vi "Uncert Table Layout.vi"(11 "Uncert In":dbl[][](array[numeric])) -> (3 "Uncert Table":string[][](array[string]))   [LabVIEW 2014]
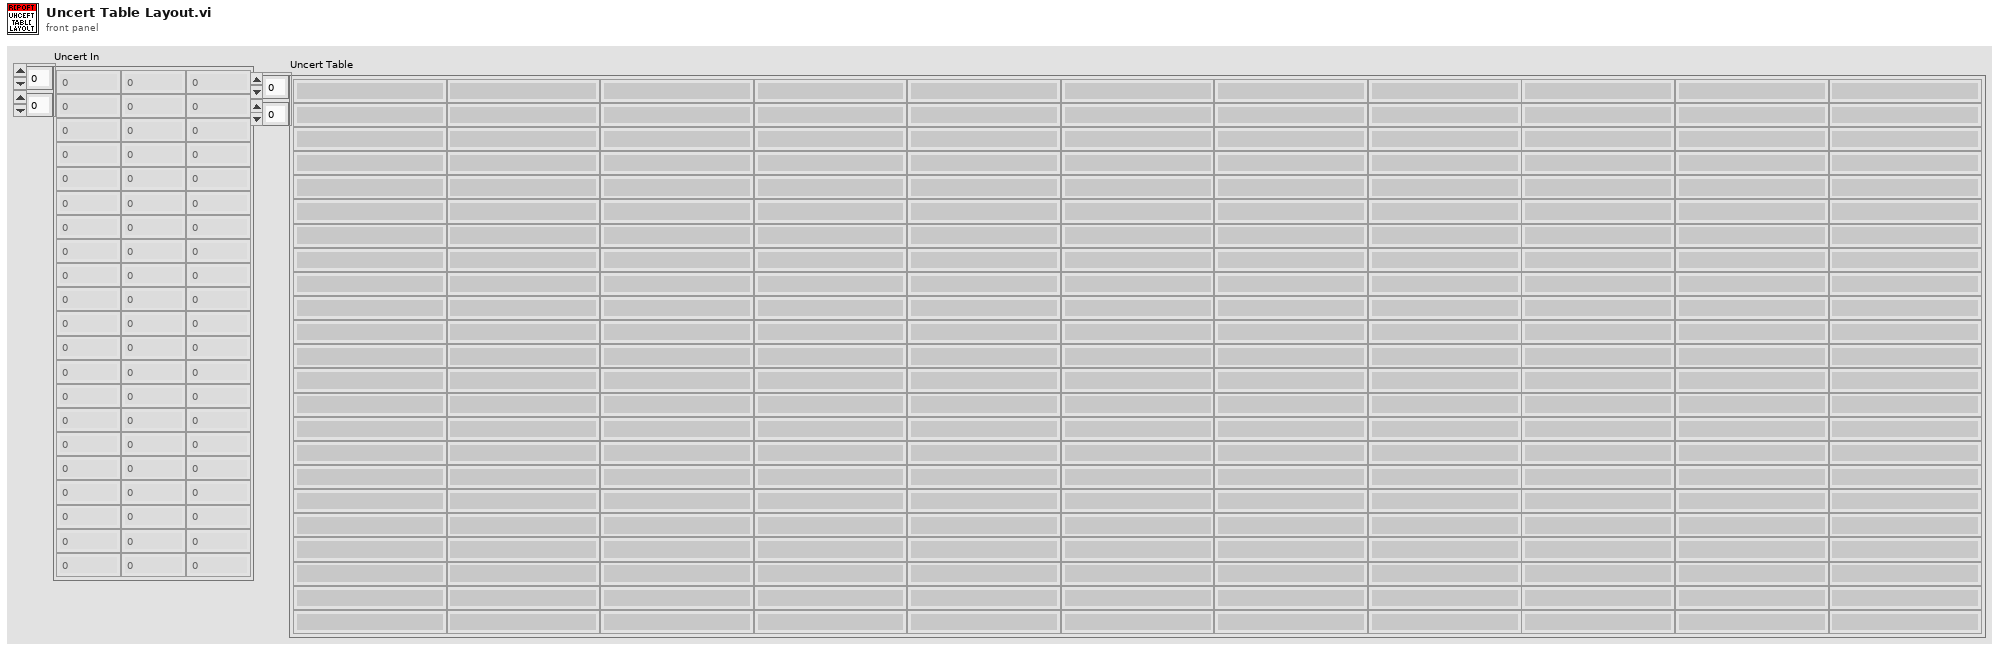
[diagram p1: front panel]
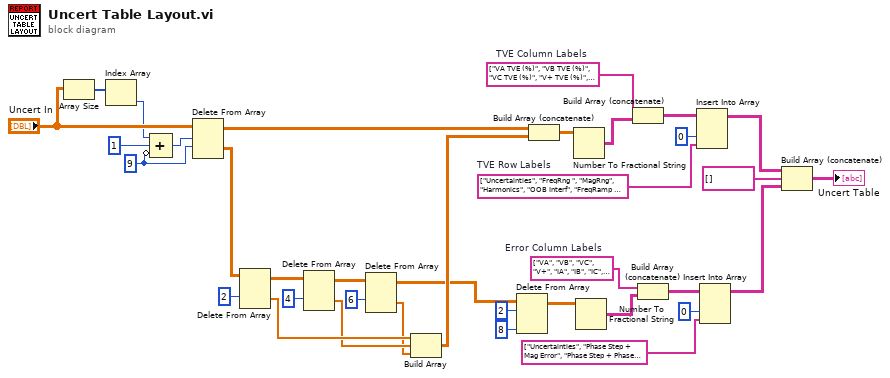
[diagram p0: block diagram]
diagram:
  w18 = string[] ["VA TVE (%)", "VB TVE (%)", "VC TVE (%)", "V+ TVE (%)", "IA TVE (%)", "IB TVE (%)", "IC TVE (%)", "I+ TVE (%)", "Freq (Hz)", "ROCOF (Hz/s)"]  # TVE Column Labels
  w16 = string[] ["VA", "VB", "VC", "V+", "IA", "IB", "IC", "I+", "", ""]  # Error Column Labels
  w10 = string[] ["Uncertainties", "FreqRng ", "MagRng", "Harmonics", "OOB Interf", "FreqRamp +", "FreqRamp -", "Mod Phase", "Mod Ampl", "Phase Step + ", "Phase Step -", "Mag Step +", "Mag Step -"]  # TVE Row Labels
  w32 = 9 ("index (row)")
  n1 = Array Size(array="Uncert In") -> (size(s)=w35:i32[])
  n2 = Index Array(array=w35) -> (element=w34:i32)  [unwired: 1 in]
  n3 = Compound Arithmetic op=ADD(w34, 1 ("value"), invert w32) -> (w31:i32)
  n4 = Delete From Array(array="Uncert In", length=w31, index (row)=w32) -> (deleted portion=w30:dbl[][], array with subset deleted=w21:dbl[][])  [unwired: 1 in]
  n5 = Delete From Array(array=w30, index (row)=2) -> (deleted portion=w24:dbl[], array with subset deleted=w28:dbl[][])  [unwired: 2 in]
  n6 = Delete From Array(array=w28, index (row)=4) -> (deleted portion=w23:dbl[], array with subset deleted=w26:dbl[][])  [unwired: 2 in]
  n7 = Delete From Array(array=w26, index (row)=6) -> (deleted portion=w22:dbl[], array with subset deleted=w4:dbl[][])  [unwired: 2 in]
  n8 = Build Array(w24, w23, w22) -> (w20:dbl[][])
  n9 = Delete From Array(array=w4, length=2, index (col)=8 ("disabled index (col)")) -> (array with subset deleted=w1:dbl[][])  [unwired: 1 in, 1 out]
  n10 = Build Array (concatenate)(w21, w20) -> (w19:dbl[][])
  n11 = Number To Fractional String(number=w19) -> (F-format string=w17:string[][])  [unwired: 3 in]
  n12 = Number To Fractional String(number=w1) -> (F-format string=w15:string[][])  [unwired: 3 in]
  n13 = Build Array (concatenate)(w18, w17) -> (w11:string[][])
  n14 = Build Array (concatenate)(w16, w15) -> (w14:string[][])
  n15 = Insert Into Array(array=w11, index (col)=0 ("disabled index (col)"), new element=w10) -> (w8:string[][])  [unwired: 1 in]
  n16 = Insert Into Array(array=w14, index (col)=0 ("disabled index (col)"), new element=string[] ["Uncertainties", "Phase Step + Mag Error", "Phase Step + Phase Error", "Phase Step - Mag Error", "Phase Step - Phase Error", "Mag Step + Mag Error", "Mag Step + Phase Error", "Mag Step - Mag Error", "Mag Step - Phase Error"] ("Error Row Labels")) -> (w6:string[][])  [unwired: 1 in]
  n17 = Build Array (concatenate)(w8, string[] [], w6) -> (→"Uncert Table":string[][])
